vi "User.GetUserName.vi"() -> (0 "User Name":string)   [LabVIEW 2012]
uses:
  User.Global.vi
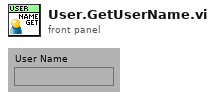
[diagram p1: front panel]
types:
  T1 = typedef "User.Info.ctl" = cluster{"ID":i32, "Name":string, "Pass":string, "Level":T2, "Del":bool}
  T2 = typedef "User.Level.ctl" = enum16{"-", "Operator", "Technician", "Administrator"}
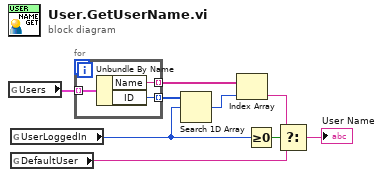
[diagram p0: block diagram]
diagram:
  n1 = global read "User.Global.vi" "Users"() -> (w6:T1[])
  n2 = global read "User.Global.vi" "UserLoggedIn"() -> (w1:i32)
  n3 = global read "User.Global.vi" "DefaultUser"() -> (w8:string)
  n4 = for {
    tunnel: w6 -> [w12] mode=indexing
    tunnel: [w11] -> w5 mode=indexing
    tunnel: [w10] -> w3 mode=indexing
    n5 = Unbundle By Name(w12) -> ("Name"=w10:string, "ID"=w11:i32)
  }
  n6 = Search 1D Array(1D array=w5, element=w1) -> (index of element=w4:i32)  [unwired: 1 in]
  n7 = Index Array(array=w3, index=w4) -> (element=w2:string)
  n8 = Greater Or Equal To 0?(x=w1) -> (x >= 0?=w7:bool)
  n9 = Select(t=w2, s=w7, f=w8) -> (s? t:f=→"User Name":string)
